vi "image2slopes.vi"(8 "error in (no error)":errorcluster, 9 "Image in":refnum<class "Image.lvclass">, 10 "HasoEngine in":refnum<class "HasoEngine.lvclass">, 11 "HasoSlopes in":refnum<class "HasoSlopes.lvclass">) -> (0 "error out":errorcluster, 1 "Image out":refnum<class "Image.lvclass">, 2 "HasoEngine out":refnum<class "HasoEngine.lvclass">, 3 "HasoSlopes out":refnum<class "HasoSlopes.lvclass">)   [LabVIEW 2018]
uses:
  <userlib>/WaveKit.lib/Controls/HasoSlopes.lvclass
  <userlib>/WaveKit.lib/Classes/Image/Image.lvclass
  <userlib>/WaveKit.lib/Classes/HasoEngine/HasoEngine.lvclass
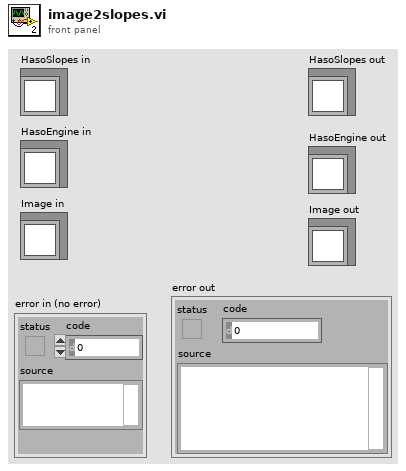
[diagram p1: front panel]
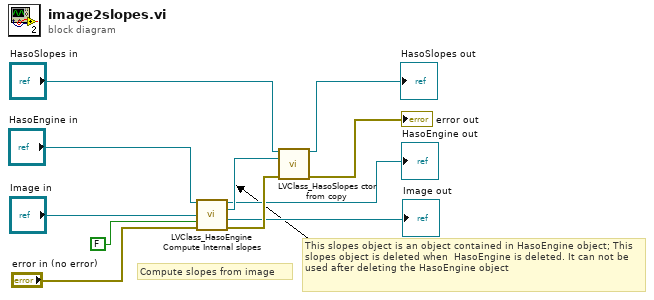
[diagram p0: block diagram]
diagram:
  # "This slopes object is an object contained in HasoEngine object; This slopes object is deleted when  HasoEngine is deleted. It can not be used after deleting the HasoEngine object"
  # "Compute slopes from image"
  n1 = call <userlib>:"LVClass_HasoEngine Compute Internal slopes.vi"("HasoEngine in"="HasoEngine in", "Image.lvclass"="Image in", "learn_from_trimmer"=FALSE, "error in (no error)"="error in (no error)") -> ("HasoEngine out"=→"HasoEngine out":refnum<class "HasoEngine.lvclass">, "HasoSlopes (dup)"=w7:refnum<class "HasoSlopes.lvclass">, "Image (dup)"=→"Image out":refnum<class "Image.lvclass">, "error out"=w4:errorcluster)  [unwired: 7 in, 1 out]
  n2 = call <userlib>:"LVClass_HasoSlopes ctor from copy.vi"("HasoSlopes in"="HasoSlopes in", "HasoSlopes copy"=w7, "error in (no error)"=w4) -> ("HasoSlopes out"=→"HasoSlopes out":refnum<class "HasoSlopes.lvclass">, "error out"=→"error out":errorcluster)  [unwired: 11 in]
